vi "7-2.vi"() -> ()   [LabVIEW 2019, in "7.lvlib"]
uses:
  7.lvlib
panel:
  out "total fuel":i32
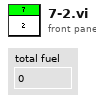
[diagram p1: front panel]
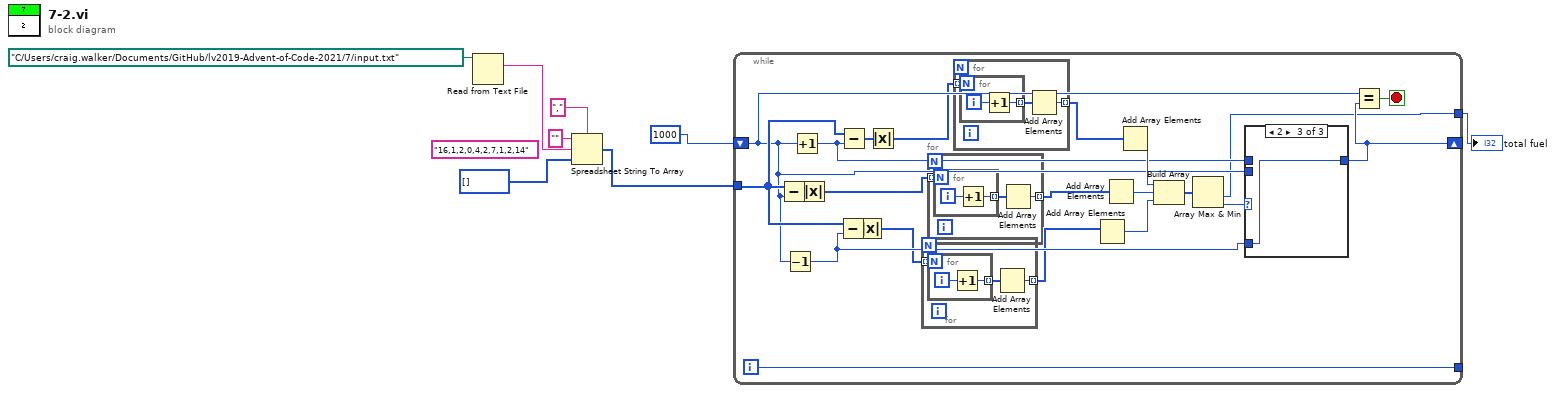
[diagram p0: block diagram]
diagram:
  (unwired) "16,1,2,0,4,2,7,1,2,14"
  n1 = Read from Text File(file (use dialog)=path "C:/Users/craig.walker/Documents/GitHub/lv2019-Advent-of-Code-2021/7/input.txt") -> (text=w4:string)  [unwired: 3 in, 3 out]
  n2 = Spreadsheet String To Array(delimiter (Tab)=",", format string="", spreadsheet string=w4, array type (2D Dbl)=i32[] []) -> (array=w5:i32[])
  n3 = while {
    tunnel: w5 -> [w29]
    shift-right: [w19] -> _
    shift-left: 1000 ("Numeric") -> [w18]
    tunnel: [w16] -> _
    tunnel: [w15] -> w1
    i -> [w16]
    stop <- w17 stop-if-true
    n4 = Subtract(x=w29, y=w18) -> (x-y=w30:i32[])
    n5 = Decrement(x=w18) -> (x-1=w20:i32)
    n6 = Increment(x=w18) -> (x+1=w21:i32)
    n7 = Absolute Value(x=w30) -> (abs(x)=w12:i32[])
    n8 = Subtract(x=w29, y=w20) -> (x-y=w27:i32[])
    n9 = Subtract(x=w29, y=w21) -> (x-y=w28:i32[])
    n10 = Absolute Value(x=w27) -> (abs(x)=w14:i32[])
    n11 = Absolute Value(x=w28) -> (abs(x)=w10:i32[])
    n12 = for {
      tunnel: [w42] -> w13 mode=indexing
      tunnel: w14 -> [w41] mode=indexing
      n13 = for {
        N: w41 -> [_]
        tunnel: [w44] -> w43 mode=indexing
        i -> [w45]
        n14 = Increment(x=w45) -> (x+1=w44:i32)
      }
      n15 = Add Array Elements(numeric array=w43) -> (sum=w42:i32)
    }
    n16 = for {
      tunnel: [w37] -> w11 mode=indexing
      tunnel: w12 -> [w36] mode=indexing
      n17 = for {
        N: w36 -> [_]
        tunnel: [w39] -> w38 mode=indexing
        i -> [w40]
        n18 = Increment(x=w40) -> (x+1=w39:i32)
      }
      n19 = Add Array Elements(numeric array=w38) -> (sum=w37:i32)
    }
    n20 = for {
      tunnel: [w32] -> w9 mode=indexing
      tunnel: w10 -> [w31] mode=indexing
      n21 = for {
        N: w31 -> [_]
        tunnel: [w34] -> w33 mode=indexing
        i -> [w35]
        n22 = Increment(x=w35) -> (x+1=w34:i32)
      }
      n23 = Add Array Elements(numeric array=w33) -> (sum=w32:i32)
    }
    n24 = Add Array Elements(numeric array=w13) -> (sum=w24:i32)
    n25 = Add Array Elements(numeric array=w11) -> (sum=w25:i32)
    n26 = Add Array Elements(numeric array=w9) -> (sum=w26:i32)
    n27 = Build Array(w26, w25, w24) -> (w23:i32[])
    n28 = Array Max & Min(array=w23) -> (min value=w15:i32, min index (indices)=w22:i32)  [unwired: 2 out]
    n29 = case shown="2" w22 {
      tunnel: w21 -> [w46 _ _]
      tunnel: [w46 w47 w48] -> w19
      tunnel: w18 -> [_ w47 _]
      tunnel: w20 -> [_ _ w48]
      frame 0, Default {
      }
      frame 1 {
      }
      frame 2 {
      }
    }
    n30 = Equal?(x=w18, y=w19) -> (x = y?=w17:bool)
  }
  "total fuel" <- w1
